vi "Dashboard Main.vi"() -> ()   [LabVIEW 2014]
uses:
  <vilib>/event_ctls.llb/eventvkey.ctl
  <vilib>/vision/Image Controls.llb/IMAQ Image.ctl
  <vilib>/Rock Robotics/WPI/Dashboard/WPI_DashboardLogging Global.vi
  <vilib>/Rock Robotics/Network Tables/SD Read Boolean Array.vi
  <vilib>/Rock Robotics/Network Tables/SD Read Number.vi
  <vilib>/Rock Robotics/Network Tables/SD Read Boolean.vi
  <vilib>/Rock Robotics/Network Tables/SD Write Number.vi
  <vilib>/Rock Robotics/Network Tables/SD Write Numeric Array.vi
  <vilib>/Utility/config.llb/Write Key (String).vi
  <vilib>/Utility/config.llb/Write Key (I32).vi
  <vilib>/Utility/config.llb/NI_LVConfig.lvlib
panel:
  in  "Camera Settings":T1={"Frame Rate"=30, "Compression"=0, "Size"=0} {"Frame Rate" scale=1.0..30.0; "Size" items=["640x480", "320x240", "160x120"]}
  in  "Camera Settings 2":T1={"Frame Rate"=30, "Compression"=30, "Size"=1} {"Frame Rate" scale=1.0..30.0; "Size" items=["640x480", "320x240", "160x120"]}
  out "Image Message 2":string="Timeout in Camera Communications"
  in  "IP1:":string="axis-top.local" caption="Address:"
  in  "DB Camera Config 2":bool
  out "Mbps 2 LED":bool
  in  "DB Camera Config":bool
  out "fps (BOT)":dbl format="%#.1g"
  out "Mbps (BOT)":dbl format="%#.1g"
  out "Mbps LED":bool
  out "Camera Image 2":T2(plugin-control)
  out "Mbps (TOP)":dbl format="%#.1g"
  out "fps (TOP)":dbl format="%#.1g"
  in  "Vision 2":u16(ring) items=["Camera Off", "USB Camera SW", "USB Camera HW", "IP Camera"]
  in  "TCP":refnum<k5>
  in  "Rec Mode":enum32{"Stop", "Record", "Playback"}(radio)
  in  "Vision":u16(ring)=3 items=["Camera Off", "USB Camera SW", "USB Camera HW", "IP Camera"]
  in  "IP2:":string="axis-bot.local" caption="Address:"
  out "Image Message":string="Timeout in Camera Communications"
  in  "Dashboard Tab":T3(tab)
  out "Clamp Latch":bool
  out "Slow and Steady":bool
  out "Gotta Go Fast":bool
  out "Clamp Position":dbl(slide) scale=0.0..2.0
  out "Lift Position":dbl(slide) scale=0.0..4.0
  in  "Manipulator Control":enum16{"Xbox", "Joystick"}(ring)
  in  "Drive Control":enum16{"Xbox", "Joystick"}(ring)
  in  "Autonomous":T4(ring)
  out "Mode":T5(ring)=enum."Disconnected"
  in  "Auto1":T6={"Direction"=enum."Forward", "Distance (ft)"=10.0}
  out "Auto0":cluster{"Numeric":dbl}
  in  "Auto6":T7={"Clockwise?"=FALSE, "Distance (ft)"=10.0, "Clockwise? 2"=FALSE}
  in  "Auto5":T8={"Direction"=enum."Forward", "Distance (ft)"=10.0, "Clockwise? 2"=FALSE}
  out "Distance":dbl
  out "MotorChart R":cluster{"Numeric":dbl, "Numeric":dbl}(graph)
  out "MotorChart L":T9(graph)
  out "MotorSliders R":cluster{"MotorSlide1":dbl, "MotorSlide2":dbl} {"MotorSlide2" scale=-1.0..1.0 scale format="%#_2e"; "MotorSlide1" scale=-1.0..1.0 scale format="%#_2e"}
  out "MotorSliders L":T10 {"MotorSlide4 2" scale=0.0..14.0 scale format="%#_2e"; "MotorSlide2" scale=-1.0..1.0 scale format="%#_2e"; "MotorSlide1" scale=-1.0..1.0 scale format="%#_2e"}
  out "JS1 Z":dbl(slide) scale=-1.0..1.0 scale format="%#_2e"
  out "Controller 1":cluster{"X":dbl, "Y":dbl}[](graph)
  out "JS1 Buttons":T11
  out "JS2 Z":dbl(slide) scale=-1.0..1.0 scale format="%#_2e"
  out "Controller 2":cluster{"X":dbl, "Y":dbl}[](graph)
  out "JS2 Buttons":T11
  out "Beam\nBreaker":bool
  out "Drive Encoders":dbl[](array[numeric])
  out "Ultrasonic":dbl format="%#_4g"
  out "Lift Encoder":dbl
  out "Limit Switches":T12
  in  "Test Slider":dbl(slide) scale=0.0..100.0 scale format="%#_3g"
  in  "On/Off":bool caption="Solenoid"
  in  "Test Name":u16(ring) items=["Select the test to run...", "Example Test", "-------------------------------", "List of tests is built in robot code.", "Replace with your own automated tests."]
  in  "Test Tree":string(tree)
  in  "Motor":cluster{"Value":dbl, "Enable":bool} {"Value" scale=-1.0..1.0 scale format="%#_3g"}
  out "Progress":T13 {"Test Progress" scale=0.0..100.0}
  in  "Rev/Fwd":cluster{"Forward":bool, "Reverse":bool}
  in  "Test Ring":u16(ring) items=["Monochrome", "Color"]
  in  "Listbox":i32(listbox)
  out "Tree":string(tree)
  out "Camera Image":T2(plugin-control)
  out "Boolean":bool
  # "1510 DASHBOARD"
  # "Recycle Rush 2015"
  # "Bottom Camera"
  # "Left"
  # "Front"
  # "Right"
  # "Battery"
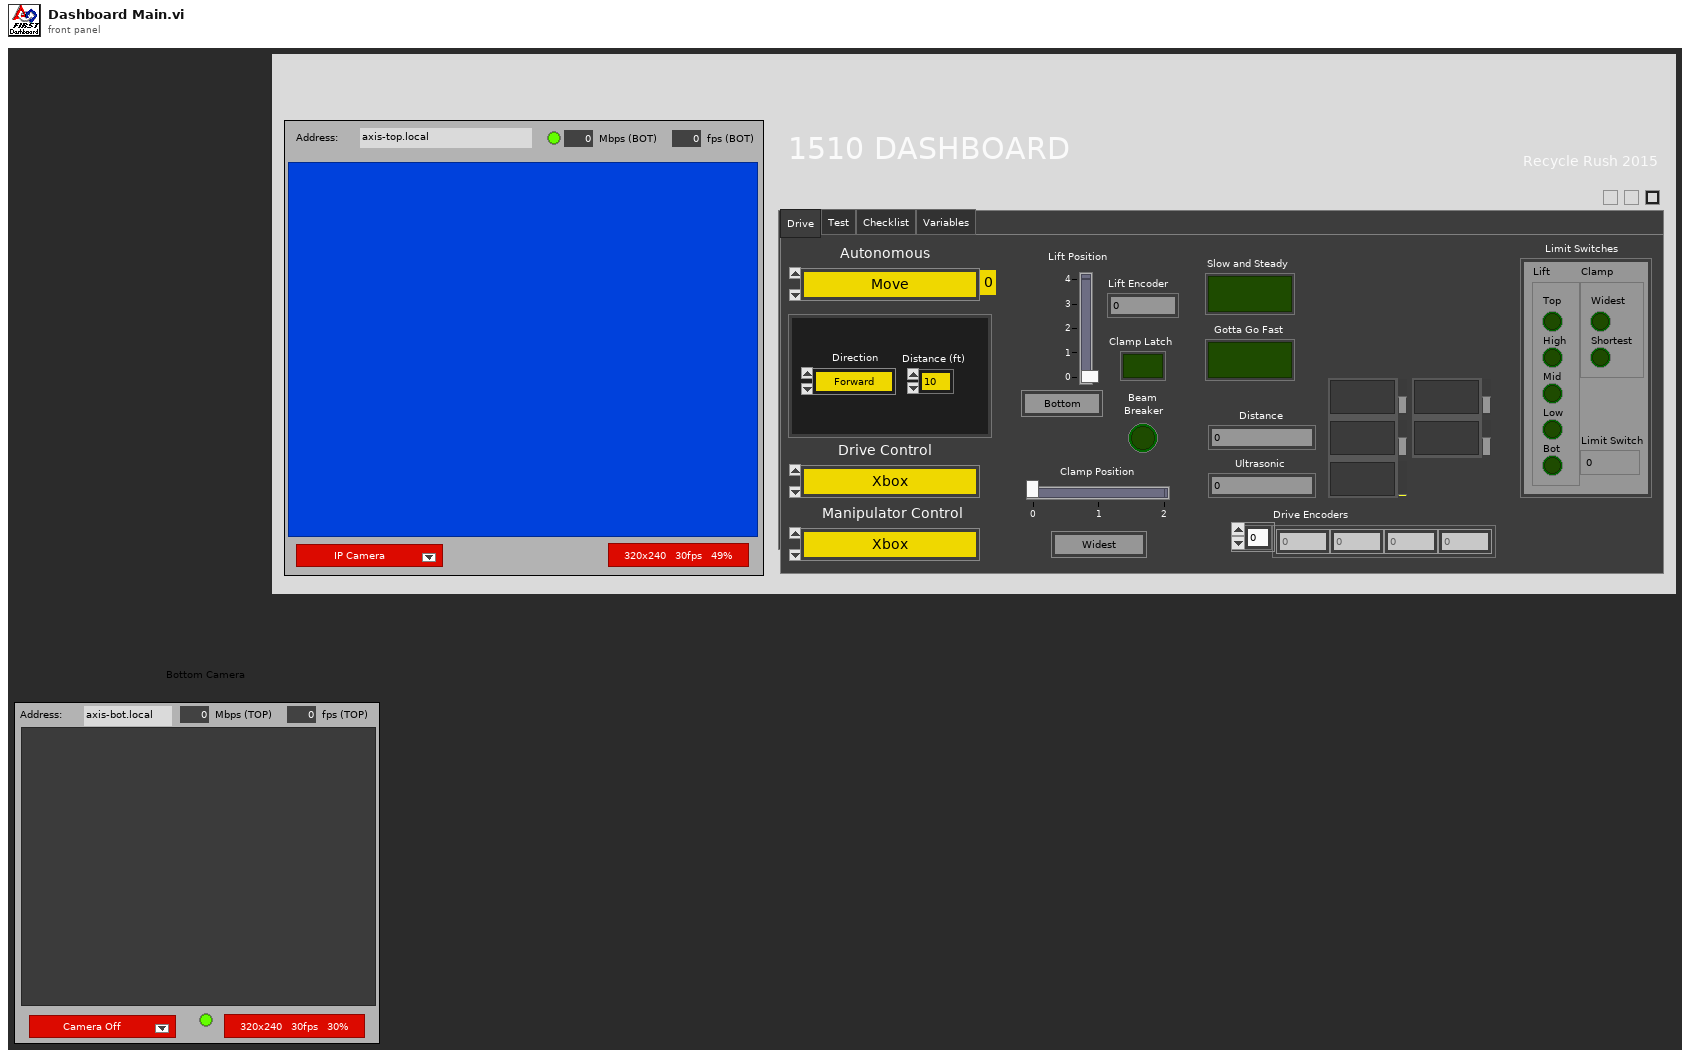
[diagram p1: front panel]
types:
  T1 = cluster{"Frame Rate":i32, "Compression":i32, "Size":u16}
  T2 = typedef "IMAQ Image.ctl" = refnum<image>
  T3 = enum32{"Drive", "Test", "Checklist", "Variables"}
  T4 = enum16{"Move", "Pick Up and Go", "Pick Up and Rotate", "3 Totes Angled", "3 Totes Strafe", "Landfill", "3 Totes Forward", "Don't Move"}
  T5 = enum8{"Tele-Op Disabled", "Tele-Op Enabled", "Auto Disabled", "Auto Enabled", "Test Disabled", "Test Enabled", "Disconnected", "No Code", "E-Stop"}
  T6 = cluster{"Direction":enum16{"Forward", "Backward", "Right", "Left"}, "Distance (ft)":dbl}
  T7 = cluster{"Clockwise?":bool, "Distance (ft)":dbl, "Clockwise? 2":bool}
  T8 = cluster{"Direction":enum16{"Forward", "Backward", "Right", "Left"}, "Distance (ft)":dbl, "Clockwise? 2":bool}
  T9 = cluster{"Numeric":dbl, "Numeric":dbl, "Battery V":dbl}
  T10 = cluster{"MotorSlide1":dbl, "MotorSlide2":dbl, "MotorSlide4 2":dbl}
  T11 = cluster{bool, bool, bool, bool, bool, bool, bool, bool, bool, bool, bool, bool}
  T12 = cluster{"Lift":cluster{"Top":bool, "High":bool, "Mid":bool, "Low":bool, "Bot":bool}, "Clamp":cluster{"Widest":bool, "Shortest":bool}, "Limit Switch":dbl}
  T13 = cluster{"Test Progress":u8, "Test Progress Text":string}
  T14 = typedef "Image Type" = u32
  T15 = enum32{"Drive", "Basic", "Custom", "Test", "Checklist", "Variables"}
  T16 = cluster{"Camera Image":refnum<vi>, "Dashboard Tab":refnum<vi>, "Boolean":refnum<vi>, "Vision":refnum<vi>, "Rec Mode":refnum<vi>, "Test Slider":refnum<vi>, "On/Off ":refnum<vi>, "Test Ring":refnum<vi>, "Rev/Fwd":refnum<vi>, "Test Name":refnum<vi>, "Motor":refnum<vi>, "Progress":refnum<vi>, "CheckList":refnum<vi>, "Tree":refnum<vi>, "Test Tree":refnum<vi>}
  T17 = cluster{"Error Strings":string, "Disable Counts":cluster{u16, u16}, "Rail Faults":cluster{u16, u16, u16}, "Robot IP":string, "DB Mode":u8, "Event Info":cluster{"Name":string, "Type":u8, "Number":u16, "Replay":u8}, "Camera Addr":string}
  T18 = cluster{"Storage":cluster{"Disk Free":u64, "RAM Block":u32, "RAM free":u32}, "CPU Utilization":cluster{"CPU % ISR":sgl, "CPU % Time Crit":sgl, "CPU % Timed Str":sgl, "CPU % High":sgl, "CPU % Above":sgl, "CPU % Normal":sgl, "CPU % Low":sgl}, "CAN":cluster{"% Bus Utilization":sgl, "Bus Off Cnt":u32, "TX_FIFO Full Cnt":u32, "Receive Error Cnt":u8, "Transmit Error Cnt":u8}, "HID":cluster{"HID Outputs":u32, "Rumble Low":u16, "Rumble High":u16}[]}
  T19 = cluster{"Status bits":cluster{"Test Mode":bool, "Autonomous":bool, "Enabled":bool, "Code Start":bool, "Brownout":bool, "Reserved 2":bool, "Reserved 3":bool, "E-Stop":bool}, "Code Trace":cluster{"Disabled":bool, "TeleOp":bool, "Auto":bool, "Test":bool}, "Controller Type":enum16{"unknown", "cRIO", "roboRio"}, "Code?":enum16{"unknown", "noCode", "code"}, "Battery V":dbl}
  T20 = cluster{"Control Bits":cluster{"TestMode":bool, "Autonomous":bool, "Enabled":bool, "FMS Present":bool, bool, bool, bool, "E-Stop":bool}, "Team Station ":u8, "Countdown":sgl, "Joystick Values":cluster{"Axes":dbl[], "Buttons":bool[], "POVs":i16[]}[]}
  T21 = cluster{"Axes":dbl[], "Buttons":bool[], "POVs":i16[]}[]
  T22 = cluster{"Boolean":bool, "Boolean":bool, "Boolean":bool, "Boolean":bool, "Boolean":bool}
  T23 = cluster{cluster{"Boolean":bool, "Boolean":bool, "Boolean":bool, "Boolean":bool, "Boolean":bool}, cluster{"Boolean":bool, "Boolean":bool}, "Numeric":dbl}
  T24 = cluster{"Axes":dbl[], "Buttons":bool[], "POVs":i16[]}
  T25 = cluster{"Buttons[0]":bool, "Buttons[1]":bool, "Buttons[2]":bool, "Buttons[3]":bool, "Buttons[4]":bool, "Buttons[5]":bool, "Buttons[6]":bool, "Buttons[7]":bool, "Buttons[8]":bool, "Buttons[9]":bool, "Buttons[10]":bool, "Buttons[11]":bool}
  T26 = typedef "NI_LVConfig.lvlib/Config Data RefNum.ctl" = refnum<k1>
  T27 = cluster{"Operation":enum16{"Update", "Clear"}, "Color Box":u32}[]
  T28 = typedef "eventvkey.ctl" = enum16{"ASCII", "Enter", "Return", "Shift", "Ctrl", "Alt", "Cmd", "Opt", "Caps", "NumLock", "Clear", "Break", "Up", "Down", "Left", "Right", "Insert", "Delete", "Home", "End", "PageUp", "PageDown", "Escape", "Help", "Pause", "ScrollLock", "F1", "F2", "F3", "F4", "F5", "F6", "F7", "F8", "F9", "F10", "F11", "F12", "F13", "F14", "F15", "F16", "F17", "F18", "F19", "F20", "F21", "F22", "F23", "F24", "Play", "VolumeUp", "VolumeDown", "Mute", "Two Byte Char"}
  T29 = cluster{"Image Size":bool, "Image Type":bool, "Pixel Value":bool, "ROI Information":bool, "Zoom Factor":bool}
  T30 = enum8{"Enabled", "Disabled", "Disabled and Grayed Out"}
  T31 = cluster{"Operation":enum16{"Update", "Clear"}, "Color Box":u32}
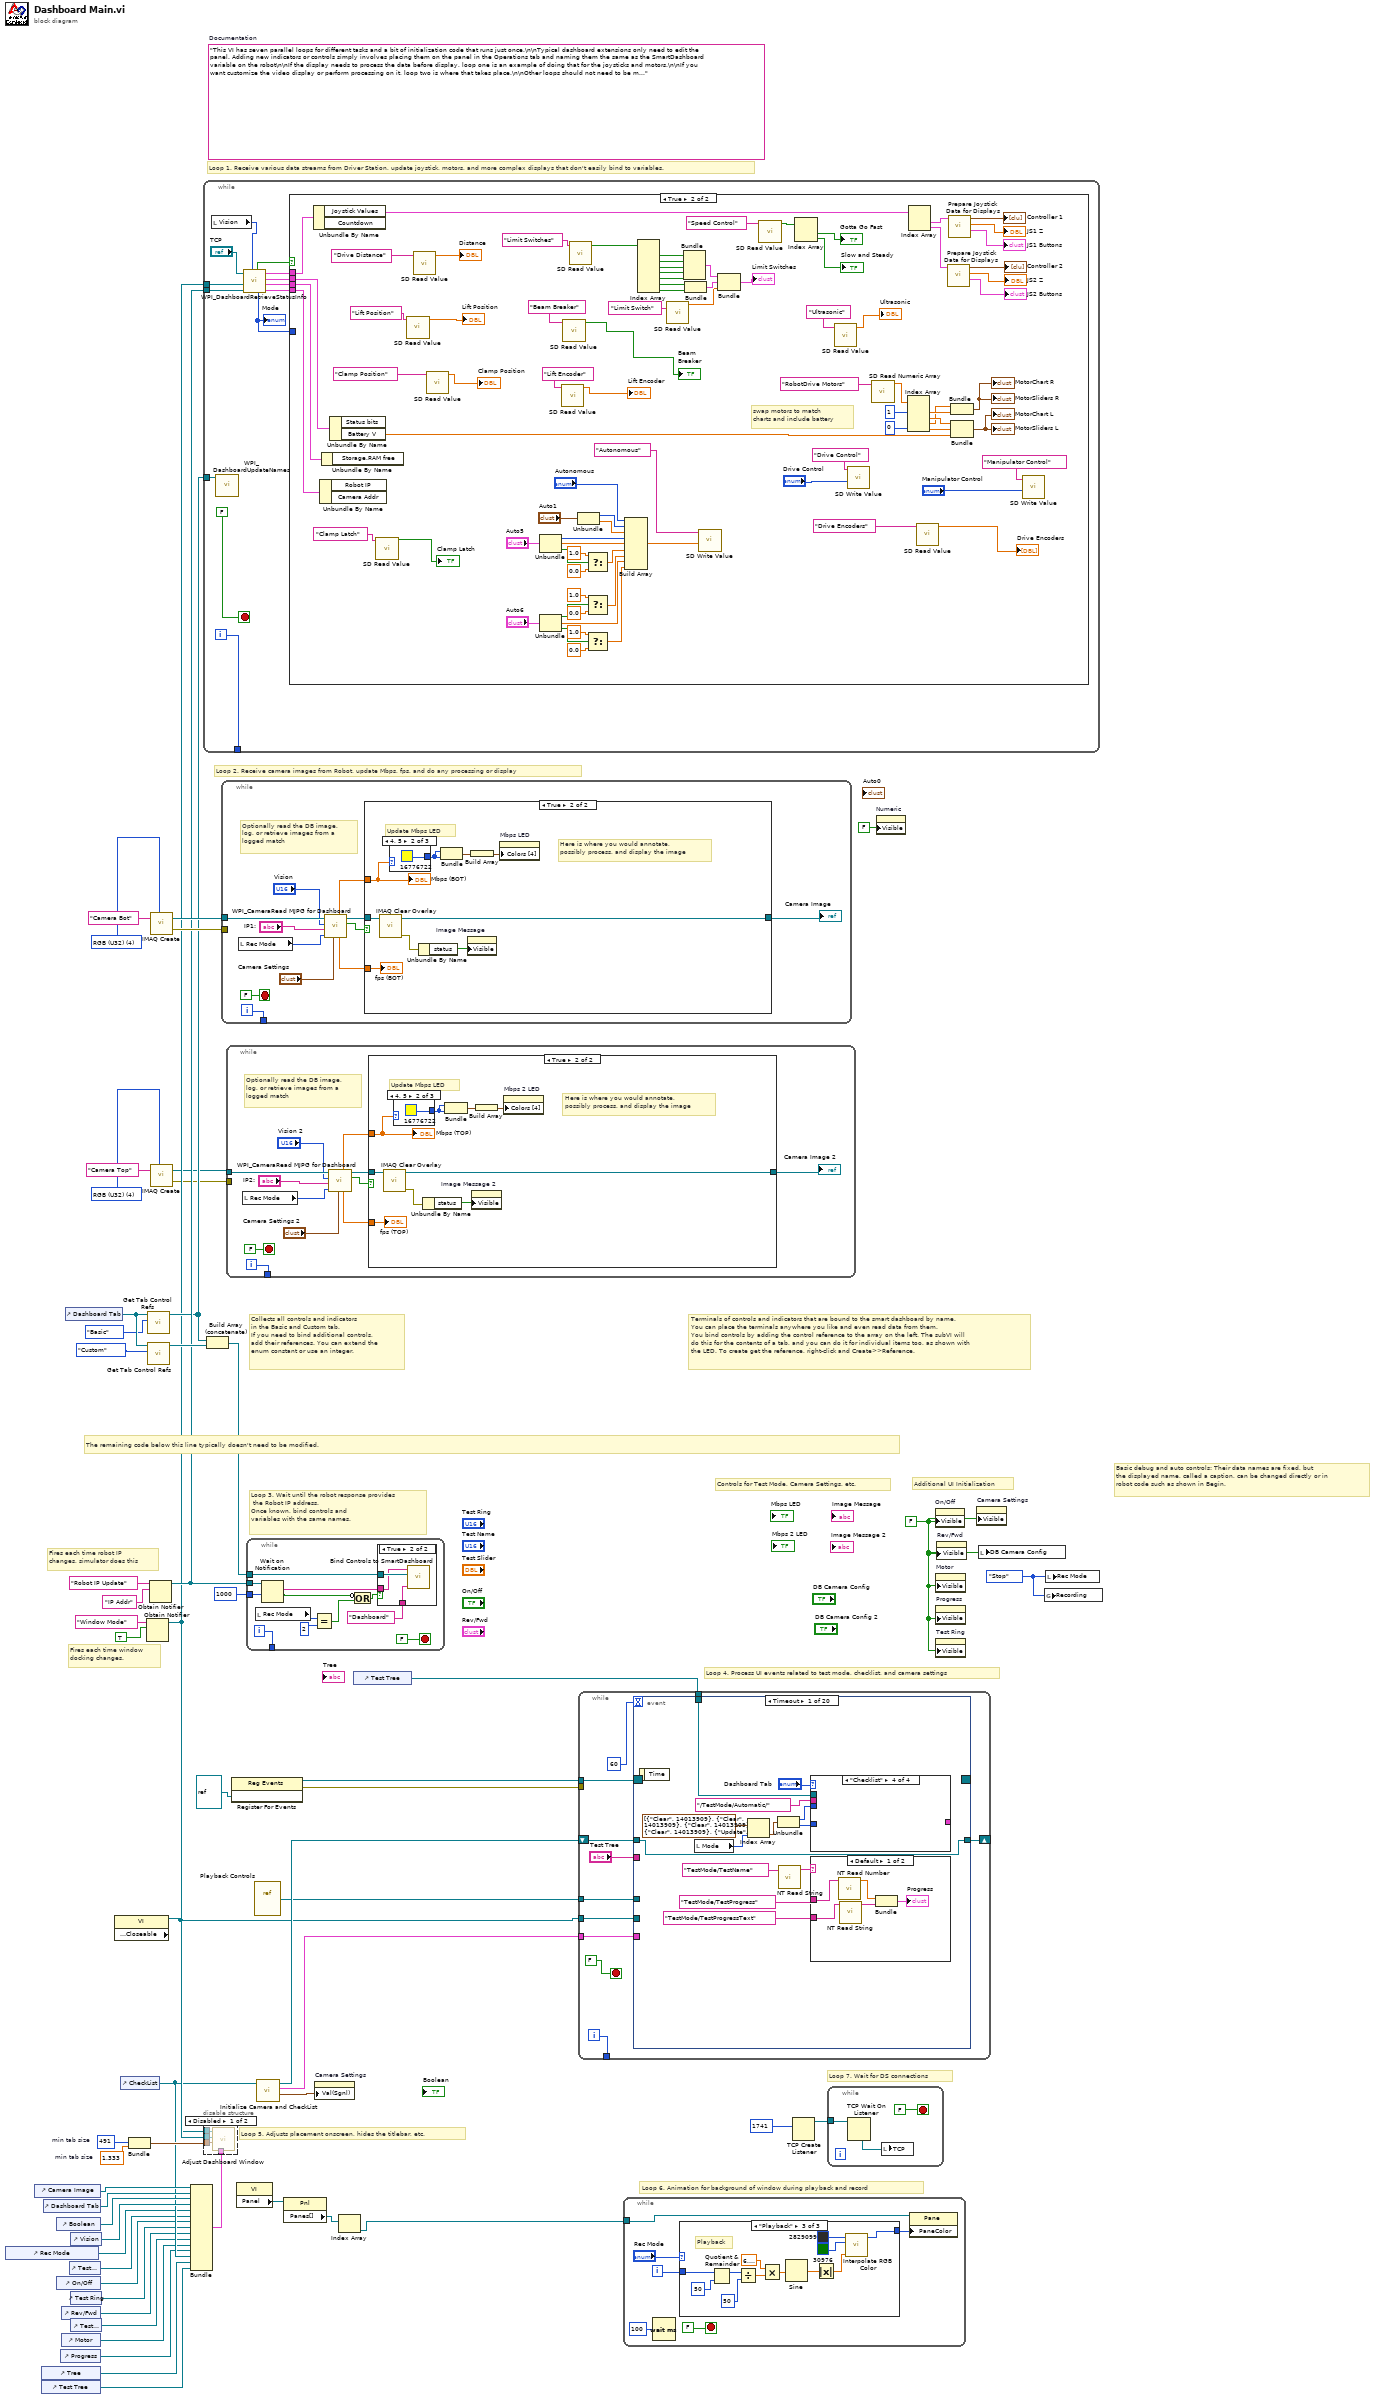
[diagram p0: block diagram]
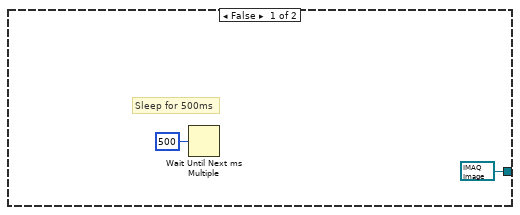
[diagram p2: hidden frame]
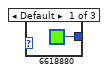
[diagram p3: hidden frame]
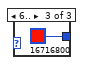
[diagram p4: hidden frame]
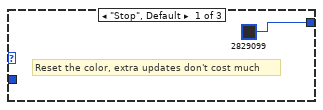
[diagram p7: hidden frame]
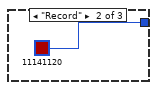
[diagram p8: hidden frame]
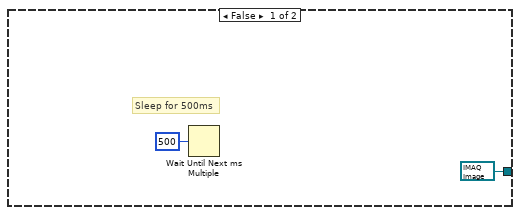
[diagram p10: hidden frame]
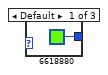
[diagram p11: hidden frame]
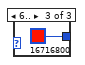
[diagram p12: hidden frame]
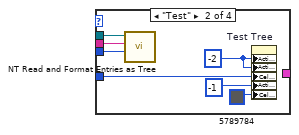
[diagram p14: hidden frame]
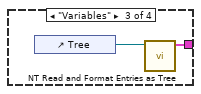
[diagram p15: hidden frame]
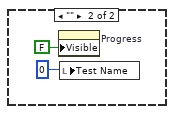
[diagram p16: hidden frame]
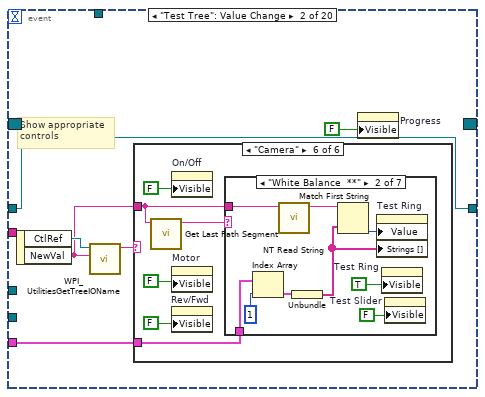
[diagram p17: hidden frame]
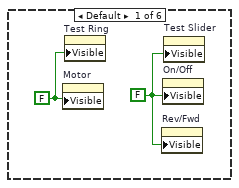
[diagram p18: hidden frame]
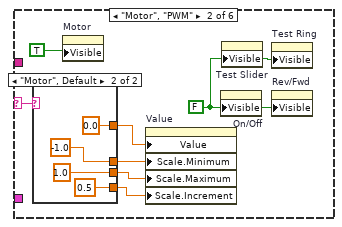
[diagram p19: hidden frame]
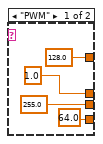
[diagram p20: hidden frame]
diagram:
  w4 = T14 4 items=["Grayscale (U8)", "Grayscale (I16)", "Grayscale (SGL)", "Complex (CSG)", "RGB (U32)", "HSL (U32)", "RGB (U64)"] ("Image Type")
  w29 = 491  # min tab size
  w28 = 1.333  # min tab size
  w37 = enum32{"Stop", "Record", "Playback"}."Stop" ("Rec Mode")
  w11 = FALSE ("Visible")
  (unwired) "This VI has seven parallel loops for different tasks and a bit of initialization code that runs just once.\n\nTypical dashboard extensions only need to edit the panel. Adding new indicators or controls simply involves placing them on the panel in the Operations tab and naming them the same as the SmartDashboard variable on the robot\n\nIf the display needs to process the data before display, loop one is an example of doing that for the joysticks and motors.\n\nIf you want customize the video display or perform processing on it, loop two is where that takes place.\n\nOther loops should not need to be modified. They are pretty standard, and document the task they perform."  # Documentation
  w57 = T14 4 items=["Grayscale (U8)", "Grayscale (I16)", "Grayscale (SGL)", "Complex (CSG)", "RGB (U32)", "HSL (U32)", "RGB (U64)"] ("Image Type")
  # "Loop 7. Wait for DS connections"
  # "Basic debug and auto controls: Their data names are fixed, but\nthe displayed name, called a caption, can be changed directly or in\nrobot code such as shown in Begin."
  # "Controls for Test Mode, Camera Settings, etc."
  # "Additional UI Initialization"
  # "Loop 6. Animation for background of window during playback and record"
  # "Fires each time robot IP\nchanges, simulator does this"
  # "Fires each time window\ndocking changes."
  # "Collects all controls and indicators\nin the Basic and Custom tab.\nIf you need to bind additional controls,\nadd their references. You can extend the\nenum constant or use an integer."
  # "The remaining code below this line typically doesn't need to be modified."
  # "Loop 4. Process UI events related to test mode, checklist, and camera settings"
  # "Terminals of controls and indicators that are bound to the smart dashboard by name.\nYou can place the terminals anywhere you like and even read data from them.\nYou bind controls by adding the control reference to the array on the left. The subVI will\ndo this for the contents of a tab, and you can do it for individual items too, as shown with\nthe LED. To create get the reference, right-click and Create>>Reference."
  # "Loop 3. Wait until the robot response provides\n the Robot IP address.\nOnce known, bind controls and\nvariables with the same names."
  # "Loop 5. Adjusts placement onscreen, hides the titlebar, etc."
  # "Loop 1. Receive various data streams from Driver Station, update joystick, motors, and more complex displays that don't easily bind to variables."
  # "Loop 2. Receive camera images from Robot, update Mbps, fps, and do any processing or display"
  n1 = control-ref of="Rec Mode"() -> (w17:refnum<vi>)
  n2 = control-ref of="Camera Image"() -> (w32:refnum<vi>)
  n3 = control-ref of="Tree"() -> (w21:refnum<vi>)
  n4 = control-ref of="Test Tree"() -> (w20:refnum<vi>)
  n5 = control-ref of="Dashboard Tab"() -> (w31:refnum<vi>)
  n6 = control-ref of="Boolean"() -> (w26:refnum<vi>)
  n7 = control-ref of="On/Off"() -> (w15:refnum<vi>)
  n8 = control-ref of="Progress"() -> (w12:refnum<vi>)
  n9 = control-ref of="Rev/Fwd"() -> (w13:refnum<vi>)
  n10 = control-ref of="Motor"() -> (w18:refnum<vi>)
  n11 = control-ref of="Dashboard Tab"() -> (w35:refnum<vi>)
  n12 = control-ref of="Test Slider"() -> (w16:refnum<vi>)
  n13 = control-ref of="Vision"() -> (w30:refnum<vi>)
  n14 = control-ref of="Test Ring"() -> (w14:refnum<vi>)
  n15 = control-ref of="Test Name"() -> (w19:refnum<vi>)
  n16 = property class="VI" props=["Front Panel.Closeable"]() -> (reference out=w36:refnum<vi>)  [unwired: 2 in, 2 out]
  n17 = control-ref of="CheckList"() -> (w22:refnum<vi>)
  n18 = Bundle("min tab size"=w29, "min tab size"=w28) -> (w27:cluster{"min tab size":i32, "min tab size":dbl})  [unwired: 1 in]
  n19 = Obtain Notifier(name (unnamed)="Window Mode", notification data type=TRUE) -> (notifier out=w8:refnum<notifier>)  [unwired: 2 in, 2 out]
  n20 = call <vilib>:"Get Tab Control Refs.vi"("Page Index"=T15."Basic" ("Dashboard Tab"), "TabControl in"=w35) -> ("ControlsOnPage"=w9:refnum<vi>[])  [unwired: 9 in]
  n21 = call <vilib>:"Get Tab Control Refs.vi"("Page Index"=T15."Custom" ("Dashboard Tab"), "TabControl in"=w35) -> ("ControlsOnPage"=w34:refnum<vi>[])  [unwired: 9 in]
  n22 = Obtain Notifier(name (unnamed)="Robot IP Update", notification data type="IP Addr" ("name (unnamed)")) -> (notifier out=w10:refnum<notifier>)  [unwired: 2 in, 2 out]
  n23 = call "IMAQ Create"("Image Name"="Camera Bot", "Image Type"=w57) -> ("New Image"=w55:T2, "error out"=w54:errorcluster)  [unwired: 2 in, 1 out]
  n24 = call "IMAQ Create"("Image Name"="Camera Top", "Image Type"=w4) -> ("New Image"=w3:T2, "error out"=w2:errorcluster)  [unwired: 2 in, 1 out]
  n25 = Bundle("Camera Image"=w32, "Dashboard Tab"=w31, "Boolean"=w26, "Vision"=w30, "Rec Mode"=w17, "Test Slider"=w16, "On/Off"=w15, "Test Ring"=w14, "Rev/Fwd"=w13, "Test Name"=w19, "Motor"=w18, "Progress"=w12, "CheckList"=w22, "Tree"=w21, "Test Tree"=w20) -> (w23:T16)  [unwired: 1 in]
  n26 = while {
    tunnel: [w69] -> _
    tunnel: w10 -> [w63]
    tunnel: w9 -> [w62]
    tunnel: w8 -> [w58]
    i -> [w69]
    stop <- FALSE stop-if-true
    n27 = local read "Vision"() -> (w60:u16)
    n28 = call <vilib>:"WPI_DashboardUpdateNames.vi"("Controls on Tab"=w62) -> ()  [unwired: 11 in]
    n29 = call <vilib>:"WPI_DashboardRetrieveStatusInfo.vi"("Vision"=w60, "Binding Refnum"=w63, "Window Mode Notifier"=w58, "TCP Cnx"="TCP") -> ("Power and Errors"=w64:T17, "Robot Metrics"=w67:T18, "Status Info"=w68:T19, "Control Info"=w65:T20, "Robot Mode"=w61:T5, "Process?"=w66:bool)  [unwired: 2 in]
    "Mode" <- w61
    n30 = case shown="True" w66 {
      tunnel: w68 -> [_ w155]
      tunnel: w67 -> [_ w154]
      tunnel: w65 -> [_ w153]
      tunnel: w64 -> [_ w152]
      tunnel: w61 -> [_ _]
      frame False {
      }
      frame True {
        # "swap motors to match\ncharts and include battery"
        n31 = Unbundle By Name(w153) -> ("Joystick Values"=w140:T21)  [unwired: 1 out]
        n32 = Unbundle By Name(w152) -> ()  [unwired: 2 out]
        n33 = Unbundle By Name(w154) -> ()  [unwired: 1 out]
        n34 = Unbundle By Name(w155) -> ("Battery V"=w141:dbl)  [unwired: 1 out]
        n35 = call-poly <vilib>:"SD Read Value.vi"("Name"="Clamp Latch") -> ("Boolean"=→"Clamp Latch":bool)  [unwired: 8 in, 2 out]
        n36 = call-poly <vilib>:"SD Read Value.vi"("Name"="Lift Position") -> ("Numeric"=→"Lift Position":dbl)  [unwired: 8 in, 2 out]
        n37 = call-poly <vilib>:"SD Read Value.vi"("Name"="Drive Distance") -> ("Numeric"=→"Distance":dbl)  [unwired: 8 in, 2 out]
        n38 = call-poly <vilib>:"SD Read Value.vi"("Name"="Clamp Position") -> ("Numeric"=→"Clamp Position":dbl)  [unwired: 8 in, 2 out]
        n39 = Unbundle("Auto5") -> ("Direction"=w85:enum16{"Forward", "Backward", "Right", "Left"}, "Distance (ft)"=w84:dbl, "Clockwise? 2"=w78:bool)
        n40 = Unbundle("Auto6") -> ("Clockwise?"=w82:bool, "Distance (ft)"=w75:dbl, "Clockwise? 2"=w72:bool)
        n41 = call-poly <vilib>:"SD Read Value.vi"("Name"="Lift Encoder") -> ("Numeric"=→"Lift Encoder":dbl)  [unwired: 8 in, 2 out]
        n42 = call-poly <vilib>:"SD Read Value.vi"("Name"="Beam Breaker") -> ("Boolean"=→"Beam\nBreaker":bool)  [unwired: 8 in, 2 out]
        n43 = call-poly <vilib>:"SD Read Value.vi"("Name"="Limit Switches") -> ("Boolean Array"=w127:bool[])  [unwired: 8 in, 2 out]
        n44 = Unbundle("Auto1") -> ("Direction"=w88:enum16{"Forward", "Backward", "Right", "Left"}, "Distance (ft)"=w87:dbl)
        n45 = Select(t=1.0, s=w78, f=0.0) -> (s? t:f=w77:dbl)
        n46 = Select(t=1.0, s=w82, f=0.0) -> (s? t:f=w76:dbl)
        n47 = Select(t=1.0, s=w72, f=0.0) -> (s? t:f=w71:dbl)
        n48 = Build Array("Autonomous", w88, w87, w85, w84, w77, w76, w75, w71) -> (w90:dbl[])
        n49 = Index Array(array=w127) -> (element #1=w126:bool, element #2=w125:bool, element #3=w124:bool, element #4=w123:bool, element #5=w122:bool, element #6=w121:bool, element #7=w120:bool)  [unwired: 7 in]
        n50 = call-poly <vilib>:"SD Read Value.vi"("Name"="Limit Switch") -> ("Numeric"=w81:dbl)  [unwired: 8 in, 2 out]
        n51 = Bundle("Boolean"=w126, "Boolean"=w125, "Boolean"=w124, "Boolean"=w123, "Boolean"=w122) -> (w119:T22)  [unwired: 1 in]
        n52 = Bundle("Boolean"=w121, "Boolean"=w120) -> (w118:cluster{"Boolean":bool, "Boolean":bool})  [unwired: 1 in]
        n53 = call-poly <vilib>:"SD Write Value.vi"("Numeric Array"=w90, "Name"="Autonomous") -> ()  [unwired: 8 in, 2 out]
        n54 = Bundle(w119, w118, "Numeric"=w81) -> (→"Limit Switches":T23)  [unwired: 1 in]
        n55 = call-poly <vilib>:"SD Read Value.vi"("Name"="Speed Control") -> ("Boolean Array"=w100:bool[])  [unwired: 8 in, 2 out]
        n56 = Index Array(array=w100) -> (element #1=→"Gotta Go Fast":bool, element #2=→"Slow and Steady":bool)  [unwired: 2 in]
        n57 = call-poly <vilib>:"SD Read Value.vi"("Name"="Ultrasonic") -> ("Numeric"=→"Ultrasonic":dbl)  [unwired: 8 in, 2 out]
        n58 = call-poly <vilib>:"SD Write Value.vi"("Numeric"="Drive Control", "Name"="Drive Control") -> ()  [unwired: 8 in, 2 out]
        n59 = call <vilib>:"SD Read Numeric Array.vi"("Name"="RobotDrive Motors") -> ("Numeric Array"=w143:dbl[])  [unwired: 8 in, 2 out]
        n60 = Index Array(array=w143, index #1=1, index #4=0) -> (element #1=w147:dbl, element #2=w148:dbl, element #3=w146:dbl, element #4=w151:dbl)  [unwired: 2 in]
        n61 = Index Array(array=w140) -> (element #1=w139:T24, element #2=w135:T24)  [unwired: 2 in]
        n62 = call-poly <vilib>:"SD Read Value.vi"("Name"="Drive Encoders") -> ("Numeric Array"=→"Drive Encoders":dbl[])  [unwired: 8 in, 2 out]
        n63 = call "Prepare Joystick Data for Displays.vi"("Joystick Values"=w135) -> ("Buttons"=→"JS2 Buttons":T25, "Z Axis"=→"JS2 Z":dbl, "Cartesian Data"=→"Controller 2":cluster{"X axis":dbl, "X axis":dbl}[])  [unwired: 8 in]
        n64 = call "Prepare Joystick Data for Displays.vi"("Joystick Values"=w139) -> ("Buttons"=→"JS1 Buttons":T25, "Z Axis"=→"JS1 Z":dbl, "Cartesian Data"=→"Controller 1":cluster{"X axis":dbl, "X axis":dbl}[])  [unwired: 8 in]
        n65 = Bundle("Numeric"=w146, "Numeric"=w147) -> (→"MotorChart R" →"MotorSliders R":cluster{"Numeric":dbl, "Numeric":dbl})  [unwired: 1 in]
        n66 = Bundle("Numeric"=w148, "Numeric"=w151, "Battery V"=w141) -> (→"MotorChart L" →"MotorSliders L":T9)  [unwired: 1 in]
        n67 = call-poly <vilib>:"SD Write Value.vi"("Numeric"="Manipulator Control", "Name"="Manipulator Control") -> ()  [unwired: 8 in, 2 out]
      }
    }
  }
  n68 = disable-structure shown="Disabled" {
    disable-tunnel: w36 -> [w159 _]
    disable-tunnel: w27 -> [w158 _]
    disable-tunnel: w23 -> [w157 _]
    disable-tunnel: w8 -> [w156 _]
    frame Disabled {
      n69 = call "Adjust Dashboard Window.vi"("Sizing Refnums"=w157, "Size Constraints"=w158, "VI"=w159, "Notifier in"=w156) -> ()  [unwired: 8 in]
    }
    frame Enabled {
    }
  }
  n70 = Build Array (concatenate)(w9, w34) -> (w33:refnum<vi>[])
  n71 = while {
    tunnel: w55 -> [w169]
    tunnel: w54 -> [_]
    tunnel: [w170] -> _
    i -> [w170]
    stop <- FALSE stop-if-true
    # "Optionally read the DB image,\nlog, or retrieve images from a\nlogged match"
    n72 = local read "Rec Mode"() -> (w163:enum32{"Stop", "Record", "Playback"})
    n73 = call <vilib>:"WPI_CameraRead MJPG for Dashboard.vi"("Camera Settings"="Camera Settings", "Rec Mode"=w163, "Camera IP"="IP1:", "Camera Mode"="Vision", "Refnum in"=w169) -> ("Active"=w167:bool, "Refnum out"=w168:T2, "FPS"=w166:dbl, "Bandwidth (Mbps)"=w165:dbl)  [unwired: 3 in]
    n74 = case shown="True" w167 {
      tunnel: w168 -> [_ w177]
      tunnel: w165 -> [_ w176]
      tunnel: w166 -> [_ w175]
      tunnel: [T2 refnum ("Image Out") w174] -> w161
      frame False {
        # "Sleep for 500ms"
        n75 = Wait Until Next ms Multiple(millisecond multiple=u32 500) -> ()  [unwired: 1 out]
      }
      frame True {
        # "Here is where you would annotate,\npossibly process, and display the image"
        # "Update Mbps LED"
        n76 = call "IMAQ Clear Overlay"("Image"=w177) -> ("error out"=w181:errorcluster, "Image Out"=w174:T2)  [unwired: 2 in, 7 out]
        n77 = case shown="4, 5" w176 {
          tunnel: [u32 6618880 ("Color Box") u32 16776722 ("Color Box") u32 16716800 ("Color Box")] -> w178
          frame Default {
          }
          frame 4, 5 {
          }
          frame 6.. {
          }
        }
        n78 = Unbundle By Name(w181) -> ("status"=w182:bool)
        n79 = Bundle("Color Box"=w178, "Color Box"=w178) -> (w180:cluster{"Color Box":u32, "Color Box":u32})  [unwired: 1 out]
        n80 = property on="Image Message" class="Str"("Visible"=w182) -> ()  [unwired: 2 in, 2 out]
        n81 = Build Array(w180) -> (w179:cluster{"Color Box":u32, "Color Box":u32}[])
        n82 = property on="Mbps LED" class="Bool (strict)"("Colors [4]"=w179) -> ()  [unwired: 2 in, 2 out]
        "Mbps (BOT)" <- w176
        "fps (BOT)" <- w175
      }
    }
    "Camera Image" <- w161
  }
  n83 = while {
    tunnel: w3 -> [w195]
    tunnel: [w196] -> _
    tunnel: w2 -> [_]
    i -> [w196]
    stop <- FALSE stop-if-true
    # "Optionally read the DB image,\nlog, or retrieve images from a\nlogged match"
    n84 = local read "Rec Mode"() -> (w189:enum32{"Stop", "Record", "Playback"})
    n85 = call <vilib>:"WPI_CameraRead MJPG for Dashboard.vi"("Camera Settings"="Camera Settings 2", "Rec Mode"=w189, "Camera IP"="IP2:", "Camera Mode"="Vision 2", "Refnum in"=w195) -> ("Active"=w193:bool, "Refnum out"=w194:T2, "FPS"=w192:dbl, "Bandwidth (Mbps)"=w191:dbl)  [unwired: 3 in]
    n86 = case shown="True" w193 {
      tunnel: w194 -> [_ w203]
      tunnel: w191 -> [_ w202]
      tunnel: w192 -> [_ w201]
      tunnel: [T2 refnum ("Image Out") w200] -> w187
      frame False {
        # "Sleep for 500ms"
        n87 = Wait Until Next ms Multiple(millisecond multiple=u32 500) -> ()  [unwired: 1 out]
      }
      frame True {
        # "Here is where you would annotate,\npossibly process, and display the image"
        # "Update Mbps LED"
        n88 = call "IMAQ Clear Overlay"("Image"=w203) -> ("error out"=w207:errorcluster, "Image Out"=w200:T2)  [unwired: 2 in, 7 out]
        n89 = case shown="4, 5" w202 {
          tunnel: [u32 6618880 ("Color Box") u32 16776722 ("Color Box") u32 16716800 ("Color Box")] -> w204
          frame Default {
          }
          frame 4, 5 {
          }
          frame 6.. {
          }
        }
        n90 = Unbundle By Name(w207) -> ("status"=w208:bool)
        n91 = Bundle("Color Box"=w204, "Color Box"=w204) -> (w206:cluster{"Color Box":u32, "Color Box":u32})  [unwired: 1 out]
        n92 = property on="Image Message 2" class="Str"("Visible"=w208) -> ()  [unwired: 2 in, 2 out]
        n93 = Build Array(w206) -> (w205:cluster{"Color Box":u32, "Color Box":u32}[])
        n94 = property on="Mbps 2 LED" class="Bool (strict)"("Colors [4]"=w205) -> ()  [unwired: 2 in, 2 out]
        "Mbps (TOP)" <- w202
        "fps (TOP)" <- w201
      }
    }
    "Camera Image 2" <- w187
  }
  n95 = register-events(refnum<vi> refnum) -> (reference out=w41:refnum<event-registration>, error out=w40:errorcluster)  [unwired: 2 in]
  n96 = property class="VI"() -> ("Panel"=w44:refnum<vi>)  [unwired: 2 in, 2 out]
  n97 = while {
    tunnel: w33 -> [w223]
    tunnel: w10 -> [w221]
    tunnel: [w219] -> _
    tunnel: u32 1000 ("milliseconds to wait") -> [w218]
    i -> [w219]
    stop <- FALSE stop-if-true
    n98 = local read "Rec Mode"() -> (w214:enum32{"Stop", "Record", "Playback"})
    n99 = Wait on Notification(notifier=w221, timeout in ms (-1)=w218) -> (notification=w220:string, timed out?=w216:bool)  [unwired: 2 in, 2 out]
    n100 = Equal?(x=w214, y=u16 2 ("Rec Mode")) -> (x = y?=w215:bool)
    n101 = Compound Arithmetic op=OR(invert w216, w215) -> (w217:bool)
    n102 = case shown="True" w217 {
      tunnel: w223 -> [_ w226]
      tunnel: w220 -> [_ w225]
      tunnel: "Dashboard" -> [_ w224]
      frame False {
      }
      frame True {
        n103 = call <vilib>:"Bind Controls to SmartDashboard.vi"("Client Name"=w224, "Bound Control Refs"=w226, "Server IP Address"=w225) -> ()  [unwired: 9 in]
      }
    }
  }
  n104 = vi-ref "Playback Controls.vi"() -> (w42:refnum<vi>)
  n105 = call "Initialize Camera and CheckList.vi"("ListBox in"=w22) -> ("Cluster"=w48:cluster{"value":i32, "value":i32, "index":i32}, "Array"=w49:cluster{string[]}[], "File Refnum"=w47:T26)  [unwired: 8 in]
  n106 = property class="Pnl"(reference=w44) -> ("Panes[]"=w45:refnum<vi>[])  [unwired: 1 in, 2 out]
  n107 = property on="Camera Settings" class="Clust (strict)"("Val(Sgnl)"=w48) -> ()  [unwired: 2 in, 2 out]
  n108 = Index Array(array=w45) -> (element=w43:refnum<vi>)  [unwired: 1 in]
  n109 = control-ref of="Test Tree"() -> (w46:refnum<vi>)
  n110 = while {
    tunnel: w49 -> [w234]
    shift-right: [w233] -> _
    shift-left: w47 -> [w232]
    tunnel: [w231] -> _
    tunnel: w46 -> [w230]
    tunnel: w42 -> [w229]
    tunnel: w41 -> [w228]
    tunnel: w40 -> [_]
    tunnel: w36 -> [w227]
    i -> [w231]
    stop <- FALSE stop-if-true
    n111 = event shown="[0] Timeout" {
      selector: w228 -> [_ _ _ _ _ _ _ _ _ _ _ _ _ _ _ _ _ _ _ _]
      dyn-events: [_ _ _ _ _ _ _ _ _ _ _ _ _ _ _ w509 _ _ _ _] -> _
      timeout: u32 60 ("milliseconds to wait") -> [_ _ _ _ _ _ _ _ _ _ _ _ _ _ _ _ _ _ _ _]
      tunnel: w230 -> [w246 _ _ _ _ _ _ _ _ _ _ _ _ _ _ _ _ _ _ _]
      tunnel: "Test Tree" -> [_ _ _ _ _ _ _ _ _ _ w478 w486 w488 w492 w500 _ _ _ _ _]
      tunnel: w234 -> [_ w268 _ _ _ _ w405 w430 w460 w472 _ _ _ _ _ _ _ _ _ _]
      tunnel: [w242 w267 w366 w371 w379 w391 w404 w429 w453 w465 w477 w484 w487 w491 w499 w511 w525 w526 w536 w541] -> w233
      tunnel: w232 -> [w242 w267 w366 w371 w379 w391 w403 w428 w453 w465 w477 w484 w487 w491 w499 w511 w525 w526 w536 w541]
      tunnel: w229 -> [_ _ _ _ _ _ _ _ _ _ _ _ _ _ _ w512 _ w529 _ _]
      tunnel: w227 -> [_ _ _ _ _ _ _ _ _ _ _ _ _ _ _ w507 _ _ _ _]
      event Timeout {
        n112 = event-data() -> ()  [unwired: 1 in, 1 out]
        n113 = local read "Mode"() -> (w245:T5)
        n114 = Index Array(array=T27 [{"Operation"=enum."Clear", "Color Box"=14013909}, {"Operation"=enum."Clear", "Color Box"=14013909}, {"Operation"=enum."Clear", "Color Box"=14013909}, {"Operation"=enum."Clear", "Color Box"=14013909}, {"Operation"=enum."Update", "Color Box"=14013909}, {"Operation"=enum."Update", "Color Box"=16777215}, {"Operation"=enum."Clear", "Color Box"=14013909}, {"Operation"=enum."Clear", "Color Box"=14013909}, {"Operation"=enum."Clear", "Color Box"=14013909}], index=w245) -> (element=w240:T31)
        n115 = Unbundle(w240) -> ("Operation"=w239:enum16{"Update", "Clear"}, "Color Box"=w238:u32)
        n116 = call <vilib>:"NT Read String.vi"("Name"="TestMode/TestName") -> ("String"=w249:string)  [unwired: 9 in, 1 out]
        n117 = case shown="\"Checklist\"" "Dashboard Tab" {
          tunnel: w246 -> [_ w257 _ _]
          tunnel: "/TestMode/Automatic/" ("Name Pattern") -> [_ w256 _ _]
          tunnel: w239 -> [_ w255 _ _]
          tunnel: [_ _ w259 _] -> _
          tunnel: w238 -> [_ w251 _ _]
          frame "Drive" {
          }
          frame "Test" {
            w254 = -2 ("Active Item:Row Number")
            n118 = call <vilib>:"NT Read and Format Entries as Tree.vi"("Operation"=w255, "Name Pattern"=w256, "Tree Refnum"=w257) -> ()  [unwired: 7 in, 2 out]
            n119 = property on="Test Tree" class="Tree (strict)"("Active Item Row Number"=w254, "ActiveColNum"=w254, "CellBG"=w251, "Active Item Row Number"=-1 ("Active Item:Row Number"), "CellBG"=u32 5789784 ("Color Box")) -> ()  [unwired: 2 in, 2 out]
          }
          frame "Variables" {
            n120 = control-ref of="Tree"() -> (w258:refnum<vi>)
            n121 = call <vilib>:"NT Read and Format Entries as Tree.vi"("Tree Refnum"=w258) -> ("Formatted Strings"=w259:cluster{"Name":string, "Value":string}[])  [unwired: 9 in, 1 out]
          }
          frame "Checklist" {
          }
        }
        n122 = case shown="Default" w249 {
          tunnel: "TestMode/TestProgress" ("Name") -> [w261 _]
          tunnel: "TestMode/TestProgressText" ("Name") -> [w260 _]
          frame Default {
            n123 = call <vilib>:"NT Read Number.vi"("Name"=w261) -> ("Numeric"=w262:dbl)  [unwired: 9 in, 1 out]
            n124 = call <vilib>:"NT Read String.vi"("Name"=w260) -> ("String"=w263:string)  [unwired: 9 in, 1 out]
            n125 = Bundle("Numeric"=w262, "String"=w263) -> (→"Progress":cluster{"Numeric":dbl, "String":string})  [unwired: 1 in]
          }
          frame "" {
            n126 = property on="Progress" class="Clust (strict)"("Visible"=FALSE) -> ()  [unwired: 2 in, 2 out]
            n127 = local write "Test Name"(u16 0) -> ()
          }
        }
      }
      event "Test Tree": Value Change {
        # "Show appropriate\ncontrols"
        n128 = event-data() -> ("CtlRef"=w271:refnum<vi>, "NewVal"=w269:string)  [unwired: 1 in]
        n129 = call <vilib>:"WPI_UtilitiesGetTreeIOName.vi"("NewVal"=w269, "TreeControl in"=w271) -> ("I/O Name"=w272:string)  [unwired: 9 in]
        n130 = case shown="\"Camera\"" w272 {
          selector: w272 -> [_ w279 _ w297 w306 _]
          tunnel: w269 -> [_ _ w294 w296 _ w313]
          tunnel: w268 -> [_ _ _ _ _ w312]
          frame Default {
            w274 = FALSE ("Visible")
            w273 = FALSE ("Visible")
            n131 = property on="Motor" class="Clust (strict)"("Visible"=w273) -> ()  [unwired: 2 in, 2 out]
            n132 = property on="Test Ring" class="Ring (strict)"("Visible"=w273) -> ()  [unwired: 2 in, 2 out]
            n133 = property on="Rev/Fwd" class="Clust (strict)"("Visible"=w274) -> ()  [unwired: 2 in, 2 out]
            n134 = property on="On/Off" class="Bool (strict)"("Visible"=w274) -> ()  [unwired: 2 in, 2 out]
            n135 = property on="Test Slider" class="Slide (strict)"("Visible"=w274) -> ()  [unwired: 2 in, 2 out]
          }
          frame "Motor", "PWM" {
            w280 = FALSE ("Visible")
            n136 = case shown="\"Motor\", Default" w279 {
              tunnel: [1.0 ("Value") -1.0 ("Value")] -> w278
              tunnel: [255.0 ("Value") 1.0 ("Value")] -> w277
              tunnel: [128.0 ("Value") 0.0 ("Value")] -> w276
              tunnel: [64.0 ("Value") 0.5 ("Value")] -> w275
              frame "PWM" {
              }
              frame "Motor", Default {
              }
            }
            n137 = property on="Motor" class="Clust (strict)"("Visible"=TRUE) -> ()  [unwired: 2 in, 2 out]
            n138 = property on="Value" class="Slide (strict)"("Value"=w276, "Scale.Minimum"=w278, "Scale.Maximum"=w277, "Scale.Increment"=w275) -> ()  [unwired: 2 in, 2 out]
            n139 = property on="On/Off" class="Bool (strict)"("Visible"=w280) -> ()  [unwired: 2 in, 2 out]
            n140 = property on="Test Slider" class="Slide (strict)"("Visible"=w280) -> ()  [unwired: 2 in, 2 out]
            n141 = property on="Test Ring" class="Ring (strict)"("Visible"=w280) -> ()  [unwired: 2 in, 2 out]
            n142 = property on="Rev/Fwd" class="Clust (strict)"("Visible"=w280) -> ()  [unwired: 2 in, 2 out]
          }
          frame "Servo" {
            w292 = FALSE ("Visible")
            n143 = call <vilib>:"NT Read Number.vi"("Name"=w294) -> ("Numeric"=w293:dbl)  [unwired: 9 in, 1 out]
            n144 = property on="Test Slider" class="Slide (strict)"("Visible"=TRUE, "Scale.Maximum"=170.0 ("Scale.Range:Maximum")) -> ()  [unwired: 2 in, 2 out]
            n145 = local write "Test Slider"(w293) -> ()
            n146 = property on="Motor" class="Clust (strict)"("Visible"=w292) -> ()  [unwired: 2 in, 2 out]
            n147 = property on="Rev/Fwd" class="Clust (strict)"("Visible"=w292) -> ()  [unwired: 2 in, 2 out]
            n148 = property on="On/Off" class="Bool (strict)"("Visible"=w292) -> ()  [unwired: 2 in, 2 out]
            n149 = property on="Test Ring" class="Ring (strict)"("Visible"=w292) -> ()  [unwired: 2 in, 2 out]
          }
          frame "Relay", "Solenoid" {
            w295 = FALSE ("Visible")
            n150 = property on="Motor" class="Clust (strict)"("Visible"=w295) -> ()  [unwired: 2 in, 2 out]
            n151 = property on="Test Slider" class="Slide (strict)"("Visible"=w295) -> ()  [unwired: 2 in, 2 out]
            n152 = Search and Replace String(input string=w296, search string="/Value  **", replace string="/Direction") -> (result string=w302:string)  [unwired: 5 in, 3 out]
            n153 = property on="Test Ring" class="Ring (strict)"("Visible"=w295) -> ()  [unwired: 2 in, 2 out]
            n154 = call <vilib>:"NT Read String.vi"("Name"=w302) -> ("String"=w300:string)  [unwired: 9 in, 1 out]
            n155 = Equal?(x="Both directions", y=w300) -> (x = y?=w298:bool)
            n156 = Not(x=w298) -> (.not. x?=w299:bool)
            n157 = property on="Rev/Fwd" class="Clust (strict)"("Visible"=w298) -> ()  [unwired: 2 in, 2 out]
            n158 = property on="On/Off" class="Bool (strict)"("Visible"=w299, "Caption.Text"=w297) -> ()  [unwired: 2 in, 2 out]
          }
          frame "Compressor", "Digital Out" {
            w305 = FALSE ("Visible")
            # "Get direction and finish"
            n159 = property on="Motor" class="Clust (strict)"("Visible"=w305) -> ()  [unwired: 2 in, 2 out]
            n160 = property on="Test Slider" class="Slide (strict)"("Visible"=w305) -> ()  [unwired: 2 in, 2 out]
            n161 = property on="Test Ring" class="Ring (strict)"("Visible"=w305) -> ()  [unwired: 2 in, 2 out]
            n162 = property on="On/Off" class="Bool (strict)"("Visible"=TRUE, "Caption.Text"=w306) -> ()  [unwired: 2 in, 2 out]
            n163 = property on="Rev/Fwd" class="Clust (strict)"("Visible"=FALSE) -> ()  [unwired: 2 in, 2 out]
          }
          frame "Camera" {
            n164 = call <vilib>:"Get Last Path Segment.vi"("String in"=w313) -> ("String out"=w314:string)  [unwired: 10 in]
            n165 = property on="On/Off" class="Bool (strict)"("Visible"=FALSE) -> ()  [unwired: 2 in, 2 out]
            n166 = property on="Motor" class="Clust (strict)"("Visible"=FALSE) -> ()  [unwired: 2 in, 2 out]
            n167 = property on="Rev/Fwd" class="Clust (strict)"("Visible"=FALSE) -> ()  [unwired: 2 in, 2 out]
            n168 = case shown="\"White Balance  **\"" w314 {
              tunnel: w313 -> [w320 w329 w338 w347 w356 _ w362]
              tunnel: w312 -> [w318 w326 w335 w344 w353 _ _]
              frame "Size  **" {
                n169 = Index Array(array=w318) -> (element=w317:cluster{string[]})  [unwired: 1 in]
                n170 = call <vilib>:"NT Read String.vi"("Name"=w320) -> ("String"=w319:string)  [unwired: 9 in, 1 out]
                n171 = Unbundle(w317) -> (w315:string[])
                n172 = Match First String(2:w315, 3:w319) -> (0:w316:i32)  [unwired: 1 out]
                n173 = property on="Test Ring" class="Ring (strict)"("Value"=w316, "Strings []"=w315) -> ()  [unwired: 2 in, 2 out]
                n174 = property on="Test Ring" class="Ring (strict)"("Visible"=TRUE) -> ()  [unwired: 2 in, 2 out]
                n175 = property on="Test Slider" class="Slide (strict)"("Visible"=FALSE) -> ()  [unwired: 2 in, 2 out]
              }
              frame "White Balance  **" {
                n176 = Index Array(array=w326, index=1) -> (element=w327:cluster{string[]})
                n177 = call <vilib>:"NT Read String.vi"("Name"=w329) -> ("String"=w328:string)  [unwired: 9 in, 1 out]
                n178 = Unbundle(w327) -> (w324:string[])
                n179 = Match First String(2:w324, 3:w328) -> (0:w323:i32)  [unwired: 1 out]
                n180 = property on="Test Ring" class="Ring (strict)"("Value"=w323, "Strings []"=w324) -> ()  [unwired: 2 in, 2 out]
                n181 = property on="Test Ring" class="Ring (strict)"("Visible"=TRUE) -> ()  [unwired: 2 in, 2 out]
                n182 = property on="Test Slider" class="Slide (strict)"("Visible"=FALSE) -> ()  [unwired: 2 in, 2 out]
              }
              frame "Exposure  **" {
                n183 = Index Array(array=w335, index=2) -> (element=w336:cluster{string[]})
                n184 = call <vilib>:"NT Read String.vi"("Name"=w338) -> ("String"=w337:string)  [unwired: 9 in, 1 out]
                n185 = Unbundle(w336) -> (w332:string[])
                n186 = Match First String(2:w332, 3:w337) -> (0:w333:i32)  [unwired: 1 out]
                n187 = property on="Test Ring" class="Ring (strict)"("Value"=w333, "Strings []"=w332) -> ()  [unwired: 2 in, 2 out]
                n188 = property on="Test Ring" class="Ring (strict)"("Visible"=TRUE) -> ()  [unwired: 2 in, 2 out]
                n189 = property on="Test Slider" class="Slide (strict)"("Visible"=FALSE) -> ()  [unwired: 2 in, 2 out]
              }
              frame "Exposure Priority  **" {
                n190 = Index Array(array=w344, index=3) -> (element=w345:cluster{string[]})
                n191 = call <vilib>:"NT Read String.vi"("Name"=w347) -> ("String"=w346:string)  [unwired: 9 in, 1 out]
                n192 = Unbundle(w345) -> (w341:string[])
                n193 = Match First String(2:w341, 3:w346) -> (0:w342:i32)  [unwired: 1 out]
                n194 = property on="Test Ring" class="Ring (strict)"("Value"=w342, "Strings []"=w341) -> ()  [unwired: 2 in, 2 out]
                n195 = property on="Test Ring" class="Ring (strict)"("Visible"=TRUE) -> ()  [unwired: 2 in, 2 out]
                n196 = property on="Test Slider" class="Slide (strict)"("Visible"=FALSE) -> ()  [unwired: 2 in, 2 out]
              }
              frame "Color Enable  **" {
                n197 = Index Array(array=w353, index=4) -> (element=w354:cluster{string[]})
                n198 = call <vilib>:"NT Read String.vi"("Name"=w356) -> ("String"=w355:string)  [unwired: 9 in, 1 out]
                n199 = Unbundle(w354) -> (w350:string[])
                n200 = Match First String(2:w350, 3:w355) -> (0:w351:i32)  [unwired: 1 out]
                n201 = property on="Test Ring" class="Ring (strict)"("Value"=w351, "Strings []"=w350) -> ()  [unwired: 2 in, 2 out]
                n202 = property on="Test Ring" class="Ring (strict)"("Visible"=TRUE) -> ()  [unwired: 2 in, 2 out]
                n203 = property on="Test Slider" class="Slide (strict)"("Visible"=FALSE) -> ()  [unwired: 2 in, 2 out]
              }
              frame Default {
                n204 = property on="Test Ring" class="Ring (strict)"("Visible"=FALSE) -> ()  [unwired: 2 in, 2 out]
                n205 = property on="Test Slider" class="Slide (strict)"("Visible"=FALSE) -> ()  [unwired: 2 in, 2 out]
              }
              frame "Brightness  **", "Color Level  **", "Compression  **", "FPS  **", "Sharpness  **" {
                n206 = call <vilib>:"NT Read Number.vi"("Name"=w362) -> ("Numeric"=w361:dbl)  [unwired: 9 in, 1 out]
                n207 = local write "Test Slider"(w361) -> ()
                n208 = property on="Test Slider" class="Slide (strict)"("Visible"=TRUE, "Scale.Maximum"=100.0 ("Scale.Range:Maximum")) -> ()  [unwired: 2 in, 2 out]
                n209 = property on="Test Ring" class="Ring (strict)"("Visible"=FALSE) -> ()  [unwired: 2 in, 2 out]
              }
            }
          }
        }
        n210 = property on="Progress" class="Clust (strict)"("Visible"=FALSE) -> ()  [unwired: 2 in, 2 out]
      }
      event "Test Name": Mouse Enter {
        # "Populate the ring with the list of tests"
        n211 = event-data() -> ()  [unwired: 1 in, 1 out]
        n212 = call <vilib>:"NT Read String Array.vi"("Name"="TestMode/TestList") -> ("String Array"=w370:string[])  [unwired: 9 in, 1 out]
        n213 = Build Array (concatenate)("Select the test to run...", w370) -> (w369:string[])
        n214 = property on="Test Name" class="Ring (strict)"("Strings []"=w369) -> ()  [unwired: 2 in, 2 out]
      }
      event "Test Name": Value Change {
        w372 = FALSE ("Visible")
        # "Tell the robot the test name to run"
        n215 = event-data() -> ("NewVal"=w376:u16)  [unwired: 1 in]
        n216 = property on="Test Name" class="Ring (strict)"() -> ("Strings []"=w377:string[])  [unwired: 2 in, 2 out]
        n217 = local write "Progress"(T13 {"Test Progress"=0, "Test Progress Text"=""} ("Progress")) -> ()
        n218 = Index Array(array=w377, index=w376) -> (element=w375:string)
        n219 = call <vilib>:"NT Write String.vi"("String"=w375, "Name"="TestMode/TestName") -> ()  [unwired: 9 in, 1 out]
        n220 = property on="Progress" class="Clust (strict)"("Visible"=TRUE) -> ()  [unwired: 2 in, 2 out]
        n221 = property on="Motor" class="Clust (strict)"("Visible"=w372) -> ()  [unwired: 2 in, 2 out]
        n222 = property on="Test Slider" class="Slide (strict)"("Visible"=w372) -> ()  [unwired: 2 in, 2 out]
        n223 = property on="On/Off" class="Bool (strict)"("Visible"=w372) -> ()  [unwired: 2 in, 2 out]
        n224 = property on="Rev/Fwd" class="Clust (strict)"("Visible"=w372) -> ()  [unwired: 2 in, 2 out]
        n225 = property on="Test Ring" class="Ring (strict)"("Visible"=w372) -> ()  [unwired: 2 in, 2 out]
      }
      event "Listbox": Double Click {
        # "Shift clears all"
        # "Update symbols on the listbox"
        n226 = event-data() -> ("PlatMods.Shift"=w380:bool, "Row"=w382:i32)  [unwired: 1 in]
        n227 = case shown="True" w380 {
          tunnel: w382 -> [w386 _]
          tunnel: 1 -> [w385 _]
          frame False {
            n228 = property on="Listbox" class="LstBox (strict)"() -> ("Item Symbols"=w384:i32[])  [unwired: 2 in, 2 out]
            n229 = Replace Array Subset(array=w384, new element=w385, index=w386) -> (w383:i32[])
            n230 = property on="Listbox" class="LstBox (strict)"("Item Symbols"=w383) -> ()  [unwired: 2 in, 2 out]
          }
          frame True {
            w387 = 0 ("Top Row")
            n231 = property on="Listbox" class="LstBox (strict)"() -> ("Number of Rows"=w389:u32)  [unwired: 2 in, 2 out]
            n232 = Initialize Array(0, w389) -> (w388:i32[])
            n233 = property on="Listbox" class="LstBox (strict)"("Top Row"=w387, "Value"=w387, "Item Symbols"=w388) -> ()  [unwired: 2 in, 2 out]
          }
        }
      }
      event "Listbox": Key Down {
        # "Update symbols on the listbox\nLeft and right keys check and uncheck"
        n234 = event-data() -> ("VKey"=w393:T28)  [unwired: 1 in]
        n235 = case shown="\"Left\", \"Right\"" w393 {
          selector: w393 -> [w398 _]
          tunnel: eventvkey."Left" ("VKey") -> [w396 _]
          frame "Left", "Right" {
            n236 = Equal?(x=w396, y=w398) -> (x = y?=w397:bool)
            n237 = Select(t=0, s=w397, f=1) -> (s? t:f=w399:i32)
            n238 = property on="Listbox" class="LstBox (strict)"() -> ("Item Symbols"=w402:i32[])  [unwired: 2 in, 2 out]
            n239 = Replace Array Subset(array=w402, new element=w399, index="Listbox") -> (w401:i32[])
            n240 = property on="Listbox" class="LstBox (strict)"("Item Symbols"=w401) -> ()  [unwired: 2 in, 2 out]
          }
          frame Default {
          }
        }
      }
      event "DB Camera Config": Value Change {
        # "Show or hide the cluster of controls, store in ini file"
        n241 = event-data() -> ("NewVal"=w406:bool)  [unwired: 1 in]
        n242 = case shown="False" w406 {
          tunnel: w405 -> [w415 _]
          tunnel: [w408 w426] -> w404
          tunnel: w403 -> [w407 w426]
          frame False {
            w422 = "Camera"
            w425 = FALSE ("Visible")
            n243 = local read "Camera Settings"() -> (w414:T1)
            n244 = Index Array(array=w415) -> (element=w418:cluster{string[]})  [unwired: 1 in]
            n245 = Unbundle(w414) -> ("Frame Rate"=w413:i32, "Compression"=w412:i32, "Size"=w416:u16)
            n246 = Unbundle(w418) -> (w417:string[])
            n247 = Index Array(array=w417, index=w416) -> (element=w411:string)
            n248 = call-poly <vilib>:"Write Key.vi"("section"=w422, "value"=w411, "key"="Size", "refnum"=w407) -> ("refnum out"=w424:T26)  [unwired: 2 in, 5 out]
            n249 = call-poly <vilib>:"Write Key.vi"("section"=w422, "value"=w413, "key"="FrameRate", "refnum"=w424) -> ("refnum out"=w423:T26)  [unwired: 1 in, 6 out]
            n250 = property on="Camera Settings" class="Clust (strict)"("Visible"=w425) -> ()  [unwired: 2 in, 2 out]
            n251 = local write "DB Camera Config"(w425) -> ()
            n252 = call-poly <vilib>:"Write Key.vi"("section"=w422, "value"=w412, "key"="Compression", "refnum"=w423) -> ("refnum out"=w409:T26)  [unwired: 1 in, 6 out]
            n253 = call <vilib>:"Close Config Data.vi"("refnum"=w409) -> ("file path"=w410:path)  [unwired: 2 in, 8 out]
            n254 = call <vilib>:"Open Config Data.vi"("configuration file path"=w410) -> ("refnum"=w408:T26)  [unwired: 8 in, 2 out]
          }
          frame True {
            n255 = property on="Camera Settings" class="Clust (strict)"("Visible"=TRUE) -> ()  [unwired: 2 in, 2 out]
          }
        }
      }
      event "DB Camera Config 2": Value Change {
        # "Show or hide the cluster of controls, store in ini file"
        n256 = event-data() -> ("NewVal"=w431:bool)  [unwired: 1 in]
        n257 = case shown="False" w431 {
          tunnel: w430 -> [w440 _]
          tunnel: [w433 w451] -> w429
          tunnel: w428 -> [w432 w451]
          frame False {
            w447 = "Camera"
            w450 = FALSE ("Visible")
            n258 = local read "Camera Settings 2"() -> (w439:T1)
            n259 = Index Array(array=w440) -> (element=w443:cluster{string[]})  [unwired: 1 in]
            n260 = Unbundle(w439) -> ("Frame Rate"=w438:i32, "Compression"=w437:i32, "Size"=w441:u16)
            n261 = Unbundle(w443) -> (w442:string[])
            n262 = Index Array(array=w442, index=w441) -> (element=w436:string)
            n263 = call-poly <vilib>:"Write Key.vi"("section"=w447, "value"=w436, "key"="Size", "refnum"=w432) -> ("refnum out"=w449:T26)  [unwired: 2 in, 5 out]
            n264 = call-poly <vilib>:"Write Key.vi"("section"=w447, "value"=w438, "key"="FrameRate", "refnum"=w449) -> ("refnum out"=w448:T26)  [unwired: 1 in, 6 out]
            n265 = local write "DB Camera Config 2"(w450) -> ()
            n266 = property on="Camera Settings 2" class="Clust (strict)"("Visible"=w450) -> ()  [unwired: 2 in, 2 out]
            n267 = call-poly <vilib>:"Write Key.vi"("section"=w447, "value"=w437, "key"="Compression", "refnum"=w448) -> ("refnum out"=w434:T26)  [unwired: 1 in, 6 out]
            n268 = call <vilib>:"Close Config Data.vi"("refnum"=w434) -> ("file path"=w435:path)  [unwired: 2 in, 8 out]
            n269 = call <vilib>:"Open Config Data.vi"("configuration file path"=w435) -> ("refnum"=w433:T26)  [unwired: 8 in, 2 out]
          }
          frame True {
            n270 = property on="Camera Settings 2" class="Clust (strict)"("Visible"=TRUE) -> ()  [unwired: 2 in, 2 out]
          }
        }
      }
      event "Camera Settings": Value Change {
        # "Update summary string when any elements of DB camera change"
        n271 = event-data() -> ("NewVal"=w464:T1)  [unwired: 1 in]
        n272 = Index Array(array=w460) -> (element=w459:cluster{string[]})  [unwired: 1 in]
        n273 = Unbundle(w464) -> ("Frame Rate"=w455:i32, "Compression"=w454:i32, "Size"=w457:u16)
        n274 = Unbundle(w459) -> (w458:string[])
        n275 = Index Array(array=w458, index=w457) -> (element=w456:string)
        n276 = Format Into String(format string="%s   %dfps   %d%%", w456, w455, w454) -> (resulting string=w461:string)  [unwired: 2 in, 1 out]
        n277 = Build Array(w461) -> (w462:string[])
        n278 = property on="DB Camera Config" class="Bool (strict)"("Strings [4]"=w462) -> ()  [unwired: 2 in, 2 out]
      }
      event "Camera Settings 2": Value Change {
        # "Update summary string when any elements of DB camera change"
        n279 = event-data() -> ("NewVal"=w476:T1)  [unwired: 1 in]
        n280 = Index Array(array=w472) -> (element=w471:cluster{string[]})  [unwired: 1 in]
        n281 = Unbundle(w476) -> ("Frame Rate"=w467:i32, "Compression"=w466:i32, "Size"=w469:u16)
        n282 = Unbundle(w471) -> (w470:string[])
        n283 = Index Array(array=w470, index=w469) -> (element=w468:string)
        n284 = Format Into String(format string="%s   %dfps   %d%%", w468, w467, w466) -> (resulting string=w473:string)  [unwired: 2 in, 1 out]
        n285 = Build Array(w473) -> (w474:string[])
        n286 = property on="DB Camera Config 2" class="Bool (strict)"("Strings [4]"=w474) -> ()  [unwired: 2 in, 2 out]
      }
      event "Motor.Enable": Value Change {
        # "When the test mode otor enable helper is set, update that\ntree row item's value"
        n287 = event-data() -> ("NewVal"=w482:bool)  [unwired: 1 in]
        n288 = Unbundle("Motor") -> ("Value"=w481:dbl)  [unwired: 1 out]
        n289 = Select(t=w481, s=w482, f=0.0) -> (s? t:f=w479:dbl)
        n290 = call <vilib>:"NT Write Number.vi"("Numeric"=w479, "Name"=w478) -> ()  [unwired: 9 in, 1 out]
      }
      event "Test Slider": Value Change {
        # "When the test mode slider helper is set, update that\ntree row item's value"
        n291 = event-data() -> ("NewVal"=w485:dbl)  [unwired: 1 in]
        n292 = call <vilib>:"NT Write Number.vi"("Numeric"=w485, "Name"=w486) -> ()  [unwired: 9 in, 1 out]
      }
      event "On/Off": Value Change {
        # "When the test mode on/off helper value is set, update that\ntree row item's value"
        n293 = event-data() -> ("NewVal"=w490:bool)  [unwired: 1 in]
        n294 = Boolean To (0,1)(Boolean=w490) -> (0, 1=w489:i16)
        n295 = call <vilib>:"NT Write Number.vi"("Numeric"=w489, "Name"=w488) -> ()  [unwired: 9 in, 1 out]
      }
      event "Rev/Fwd": Value Change {
        # "When the test mode helper value for relays is set, update that\ntree row item's value"
        n296 = event-data() -> ("NewVal.Forward"=w498:bool, "NewVal.Reverse"=w497:bool)  [unwired: 1 in]
        n297 = Boolean To (0,1)(Boolean=w498) -> (0, 1=w494:i16)
        n298 = Boolean To (0,1)(Boolean=w497) -> (0, 1=w496:i16)
        n299 = Negate(x=w496) -> (-x=w495:i16)
        n300 = Add(x=w494, y=w495) -> (x+y=w493:i16)
        n301 = call <vilib>:"NT Write Number.vi"("Numeric"=w493, "Name"=w492) -> ()  [unwired: 9 in, 1 out]
      }
      event "Test Ring": Value Change {
        # "When a test mode helper value is selected from the ring,\nset the tree item's variable to the string value"
        n302 = event-data() -> ("NewVal"=w502:u16)  [unwired: 1 in]
        n303 = property on="Test Ring" class="Ring (strict)"() -> ("Strings []"=w503:string[])  [unwired: 2 in, 2 out]
        n304 = Index Array(array=w503, index=w502) -> (element=w501:string)
        n305 = call <vilib>:"NT Write String.vi"("String"=w501, "Name"=w500) -> ()  [unwired: 9 in, 1 out]
      }
      event "Rec Mode": Value Change {
        # "Update globals for recording mode and path to read log from.\nClear when logging and let NetworkTables set path for vision to\nuse."
        n306 = event-data() -> ("NewVal"=w513:enum32{"Stop", "Record", "Playback"})  [unwired: 1 in]
        n307 = global write "WPI_DashboardLogging Global.vi" "Logging Filename"(path "") -> ()
        n308 = case shown="\"Playback\"" w513 {
          tunnel: w512 -> [_ w515 w523]
          tunnel: [_ _ w522] -> w509
          tunnel: [_ _ w521] -> _
          tunnel: w507 -> [_ _ w519]
          tunnel: cluster{i32, i32} {-250, 170} -> [_ _ w518]
          tunnel: [_ _ T29 {"Image Size"=TRUE, "Image Type"=TRUE, "Pixel Value"=TRUE, "ROI Information"=TRUE, "Zoom Factor"=FALSE} ("Image Information Shown:All Elements")] -> w505
          tunnel: [_ _ TRUE ("Zoom Factor")] -> w504
          frame Default {
          }
          frame "Stop", "Record" {
            # "Place Window too"
            n309 = invoke class="VI" method="FP.Close"(reference=w515) -> (reference out=w514:refnum<vi>)  [unwired: 2 in, 2 out]
            n310 = invoke class="VI" method="Abort VI"(reference=w514) -> ()  [unwired: 2 in, 3 out]
          }
          frame "Playback" {
            n311 = call "Open Playback Panel.vi"("Offset"=w518, "DB VI Ref"=w519, "Playback in"=w523) -> ("Playback out"=w520:refnum<vi>)  [unwired: 8 in]
            n312 = register-events(w520) -> (reference out=w522:refnum<event-registration>, error out=w521:errorcluster)  [unwired: 2 in]
          }
        }
        n313 = global write "WPI_DashboardLogging Global.vi" "Recording"(w513) -> ()
        n314 = property on="Camera Image" class="ImageControl"("Image Information Shown"=w505, "Image Information Visible"=w504) -> ()  [unwired: 2 in, 2 out]
        n315 = call <vilib>:"WPI_DashboardNT Log FieldName Cache.vi"("Operation"=enum16{"Lookup/Add", "Index", "Clear"}."Clear") -> ()  [unwired: 8 in, 3 out]
      }
      event Panel Close {
        w524 = enum32{"Stop", "Record", "Playback"}."Stop" ("Rec Mode")
        # "Playback window has been closed, abort"
        n316 = event-data() -> ()  [unwired: 1 in, 4 out]
        n317 = local write "Rec Mode"(w524) -> ()
        n318 = global write "WPI_DashboardLogging Global.vi" "Recording"(w524) -> ()
      }
      event Panel Close {
        # "Abort playback window and ourself"
        n319 = event-data() -> ()  [unwired: 1 in, 4 out]
        n320 = invoke class="VI" method="FP.Close"(reference=w529) -> (reference out=w528:refnum<vi>)  [unwired: 2 in, 2 out]
        n321 = invoke class="VI" method="Abort VI"(reference=w528) -> (error out=w527:errorcluster)  [unwired: 2 in, 2 out]
        n322 = invoke class="VI" method="Abort VI"(error in=w527) -> ()  [unwired: 2 in, 3 out]
      }
      event "Vision": Value Change {
        # "Enable/Disable Compression slider.\nHW USB is hard-coded into the camera"
        n323 = event-data() -> ("NewVal"=w535:u16)  [unwired: 1 in]
        n324 = Equal?(x=w535, y=u32 2 ("milliseconds to wait")) -> (x = y?=w533:bool)
        n325 = Select(t=T30."Disabled and Grayed Out" ("Disabled"), s=w533, f=T30."Enabled" ("Disabled")) -> (s? t:f=w530:T30)
        n326 = property on="Compression" class="Slide (strict)"("DisabledEnum"=w530) -> ()  [unwired: 2 in, 2 out]
      }
      event "Autonomous": Value Change {
        n327 = event-data() -> ("NewVal"=w542:T4)  [unwired: 1 in, 5 out]
        n328 = case shown="\"Move\", Default" w542 {
          tunnel: [w543 w546 w547 TRUE ("Visible") TRUE ("Visible") TRUE ("Visible") TRUE ("Visible") TRUE ("Visible")] -> w540
          tunnel: [TRUE ("Visible") w546 w547 w550 w552 w554 w556 w558] -> w539
          tunnel: [w543 TRUE ("Visible") w547 w550 w552 w554 w556 w558] -> w538
          tunnel: [w543 w546 TRUE ("Visible") w550 w552 w554 w556 w558] -> w537
          frame "Move", Default {
            w543 = FALSE ("Visible")
          }
          frame "Pick Up and Go" {
            w546 = FALSE ("Visible")
          }
          frame "Pick Up and Rotate" {
            w547 = FALSE ("Visible")
          }
          frame "3 Totes Angled" {
            w550 = FALSE ("Visible")
          }
          frame "3 Totes Strafe" {
            w552 = FALSE ("Visible")
          }
          frame "Landfill" {
            w554 = FALSE ("Visible")
          }
          frame "3 Totes Forward" {
            w556 = FALSE ("Visible")
          }
          frame "Don't Move" {
            w558 = FALSE ("Visible")
          }
        }
        n329 = property on="Auto0" class="Clust (strict)"("Visible"=w540) -> ()  [unwired: 2 in, 2 out]
        n330 = property on="Auto1" class="Clust (strict)"("Visible"=w539) -> ()  [unwired: 2 in, 2 out]
        n331 = property on="Auto5" class="Clust (strict)"("Visible"=w538) -> ()  [unwired: 2 in, 2 out]
        n332 = property on="Auto6" class="Clust (strict)"("Visible"=w537) -> ()  [unwired: 2 in, 2 out]
      }
    }
  }
  n333 = while {
    tunnel: w43 -> [w560]
    i -> [w563]
    stop <- FALSE stop-if-true
    n334 = Wait (ms)(milliseconds to wait=u32 100) -> ()  [unwired: 1 out]
    n335 = case shown="\"Playback\"" "Rec Mode" {
      tunnel: w563 -> [_ _ w578]
      tunnel: [u32 2829099 ("Base Color") u32 11141120 ("Target Color") w567] -> w559
      frame "Stop", Default {
        # "Reset the color, extra updates don't cost much"
      }
      frame "Record" {
      }
      frame "Playback" {
        # "Playback"
        n336 = Quotient & Remainder(x=w578, y=u32 50 ("milliseconds to wait")) -> (x-y*floor(x/y)=w574:u32)  [unwired: 1 out]
        n337 = Divide(x=w574, y=u32 50 ("milliseconds to wait")) -> (x/y=w571:dbl)
        n338 = Multiply(x=6.283185307179586, y=w571) -> (x*y=w576:dbl)
        n339 = Sine(x=w576) -> (sin(x)=w575:dbl)
        n340 = Absolute Value(x=w575) -> (abs(x)=w568:dbl)
        n341 = call "Interpolate RGB Color.vi"("Proportion"=w568, "Target Color"=u32 30976, "Base Color"=u32 2829099) -> ("Result Color"=w567:u32)  [unwired: 8 in]
      }
    }
    n342 = property class="Pane"(reference=w560, "PaneColor"=w559) -> ()  [unwired: 1 in, 2 out]
  }
  n343 = TCP Create Listener(10:u16 1741 ("timeout ms (25000)")) -> (3:w6:refnum<k5>)  [unwired: 4 in, 2 out]
  n344 = while {
    tunnel: w6 -> [w580]
    stop <- FALSE stop-if-true
    n345 = TCP Wait On Listener(11:w580) -> (4:w579:refnum<k5>)  [unwired: 3 in, 4 out]
    n346 = local write "TCP"(w579) -> ()
  }
  n347 = property on="Numeric" class="DigNum (strict)"("Visible"=FALSE) -> ()  [unwired: 2 in, 2 out]
  n348 = property on="On/Off" class="Bool (strict)"("Visible"=w11) -> ()  [unwired: 2 in, 2 out]
  n349 = property on="Motor" class="Clust (strict)"("Visible"=w11) -> ()  [unwired: 2 in, 2 out]
  n350 = property on="Progress" class="Clust (strict)"("Visible"=w11) -> ()  [unwired: 2 in, 2 out]
  n351 = property on="Test Ring" class="Ring (strict)"("Visible"=w11) -> ()  [unwired: 2 in, 2 out]
  n352 = property on="Rev/Fwd" class="Clust (strict)"("Visible"=w11) -> ()  [unwired: 2 in, 2 out]
  n353 = property on="Camera Settings" class="Clust (strict)"("Visible"=w11) -> ()  [unwired: 2 in, 2 out]
  n354 = local write "DB Camera Config"(w11) -> ()
  n355 = global write "WPI_DashboardLogging Global.vi" "Recording"(w37) -> ()
  n356 = local write "Rec Mode"(w37) -> ()
